vi "TestLookUpTable.vi"() -> ()   [LabVIEW 2011]
panel:
  out "Allowable Error in Wheel Speed":dbl
  out "Required Speed":dbl
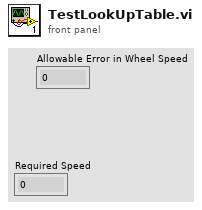
[diagram p1: front panel]
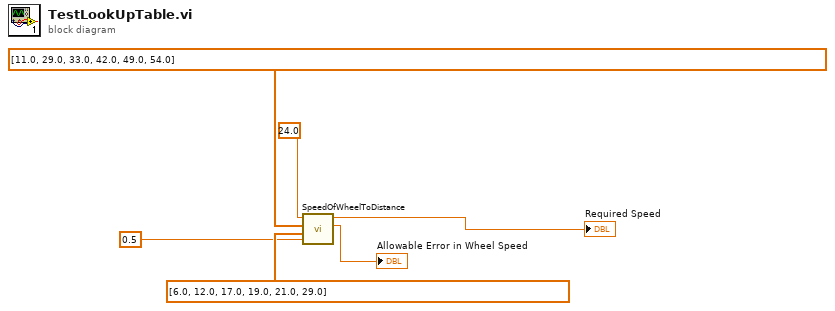
[diagram p0: block diagram]
diagram:
  n1 = call "SpeedOfWheelToDistance.vi"("Allowable Error in Distance"=0.5, "Speeds"=dbl[] [6.0, 12.0, 17.0, 19.0, 21.0, 29.0], "Distances"=dbl[] [11.0, 29.0, 33.0, 42.0, 49.0, 54.0], "Required Distance"=24.0) -> ("Allowable Error in Wheel Speed"=→"Allowable Error in Wheel Speed":dbl, "Required Speed"=→"Required Speed":dbl)  [unwired: 6 in]
